vi "Health Monitoring System(Lab_View).vi"() -> ()   [LabVIEW 2020]
panel:
  in  "PORT NAME":refnum<visa-resource-name>
  in  "Data of patient":string[][](table)
  out "Temperature":dbl(graph)
  out "Heart rate BPM":dbl(graph)
  out "Temperature":dbl(slide) scale=0.0..100.0
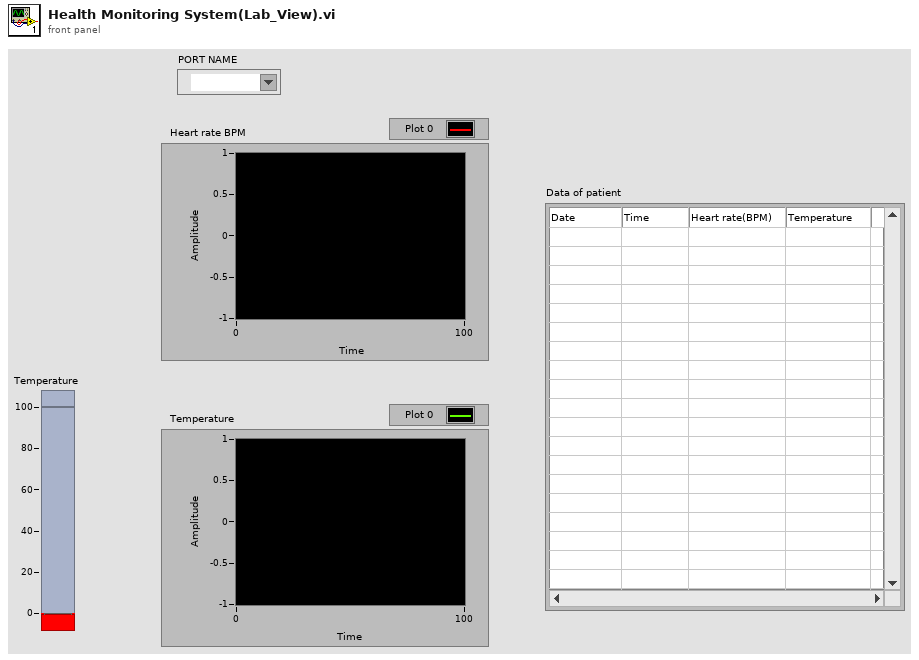
[diagram p1: front panel]
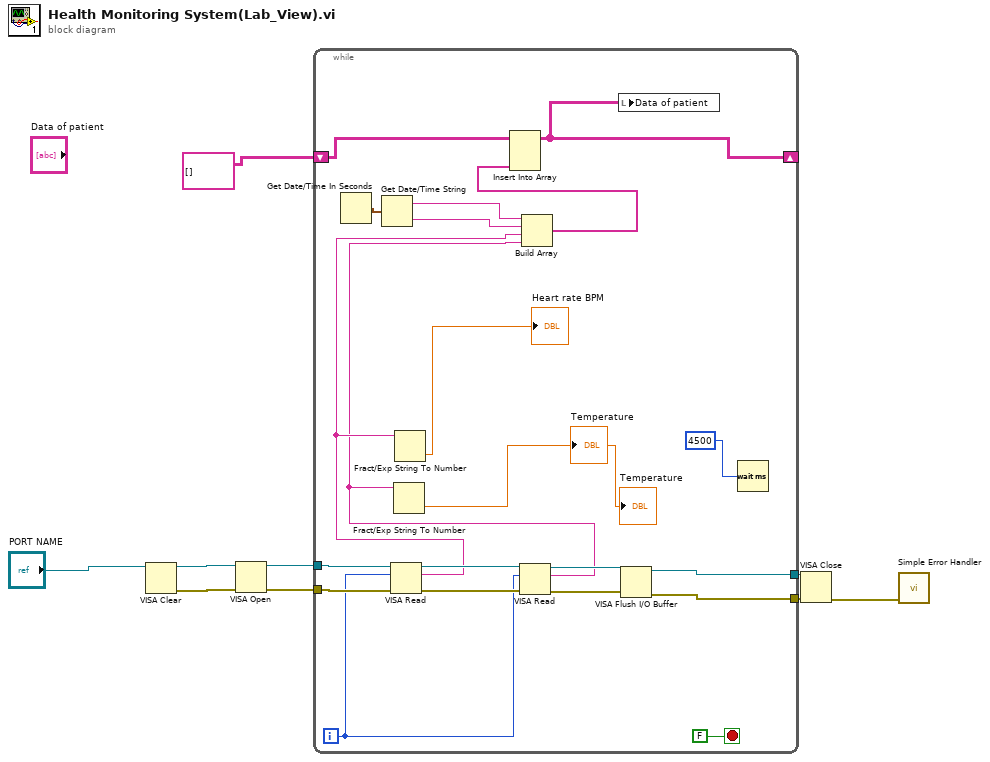
[diagram p0: block diagram]
diagram:
  n1 = VISA Clear(VISA resource name="PORT NAME") -> (VISA resource name out=w8:refnum<visa-resource-name>, error out=w9:errorcluster)  [unwired: 1 in]
  n2 = VISA Open(error in (no error)=w9, VISA resource name=w8) -> (VISA resource name=w6:refnum<visa-resource-name>, error out=w5:errorcluster)  [unwired: 3 in]
  n3 = while {
    tunnel: w6 -> [w30]
    tunnel: w5 -> [w29]
    tunnel: [w26] -> w4
    tunnel: [w25] -> w3
    shift-right: [w19] -> _
    shift-left: string[][] [] -> [w20]
    i -> [w22]
    stop <- FALSE stop-if-true
    n4 = Get Date/Time In Seconds() -> (seconds since 1Jan1904=w18:timestamp)
    n5 = Get Date/Time String(seconds (now)=w18) -> (date string=w17:string, time string=w16:string)  [unwired: 2 in]
    n6 = VISA Read(VISA resource name=w30, byte count=w22, error in (no error)=w29) -> (VISA resource name out=w28:refnum<visa-resource-name>, read buffer=w15:string, error out=w24:errorcluster)  [unwired: 1 out]
    n7 = Fract/Exp String To Number(string=w15) -> (number=→"Heart rate BPM":dbl)  [unwired: 3 in, 1 out]
    n8 = VISA Read(VISA resource name=w28, byte count=w22, error in (no error)=w24) -> (VISA resource name out=w27:refnum<visa-resource-name>, read buffer=w14:string, error out=w23:errorcluster)  [unwired: 1 out]
    n9 = Fract/Exp String To Number(string=w14) -> (number=→"Temperature" →"Temperature":dbl)  [unwired: 3 in, 1 out]
    n10 = Build Array "Build Array"(w17, w16, w15, w14) -> (w13:string[])
    n11 = Insert Into Array "Insert Into Array"(array=w20, new element=w13) -> (w19:string[][])  [unwired: 2 in]
    n12 = local write "Data of patient"(w19) -> ()
    n13 = VISA Flush I/O Buffer(VISA resource name=w27, error in (no error)=w23) -> (VISA resource name out=w26:refnum<visa-resource-name>, error out=w25:errorcluster)  [unwired: 1 in]
    n14 = Wait (ms)(milliseconds to wait=u32 4500 ("millisecond timer value")) -> ()  [unwired: 1 out]
  }
  n15 = VISA Close(VISA resource name=w4, error in (no error)=w3) -> (error out=w7:errorcluster)
  n16 = call <vilib>:"Simple Error Handler.vi"("error in (no error)"=w7) -> ()  [unwired: 4 in, 5 out]
